vi "Test Available.vi"() -> ()   [LabVIEW 2014, in "Arduino SoftwareSerial Wrapper.lvlib"]
uses:
  Arduino SoftwareSerial Wrapper.lvlib
panel:
  out "Bytes to read":u16
  out "Error Out":errorcluster
  in  "Error In":errorcluster
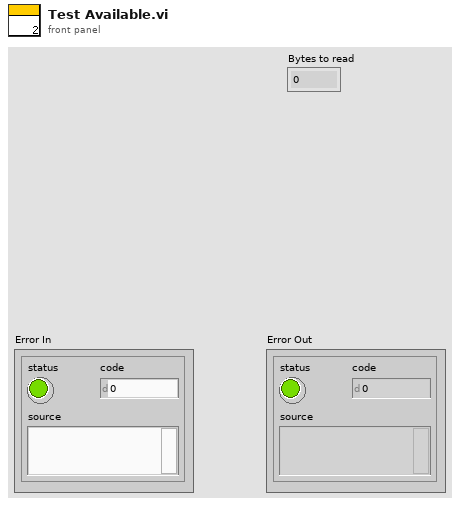
[diagram p1: front panel]
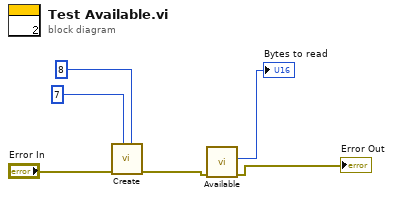
[diagram p0: block diagram]
diagram:
  n1 = call "Create.vi"("arduino RX pin"=u8 8 ("RX pin"), "arduino TX pin"=u8 7 ("RX pin"), "Error In"="Error In") -> ("Error Out"=w3:errorcluster)  [unwired: 8 in]
  n2 = call "Available.vi"("Error In"=w3) -> ("Error Out"=→"Error Out":errorcluster, "Bytes to read"=→"Bytes to read":u16)  [unwired: 9 in]
